vi "Init.vi"(11 "AllObjs[]":refnum<vi>[](array[refnum])) -> (1 "Ball Ref":cluster{refnum<vi>, "PaneColor":u32}[](array[cluster]), 2 "Array 2":refnum<vi>[](array[refnum]), 3 "Array":i32[](array[numeric]))   [LabVIEW 2014]
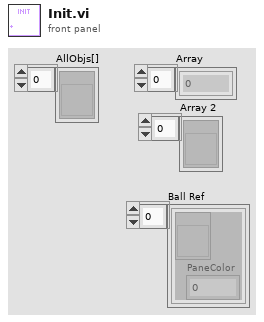
[diagram p1: front panel]
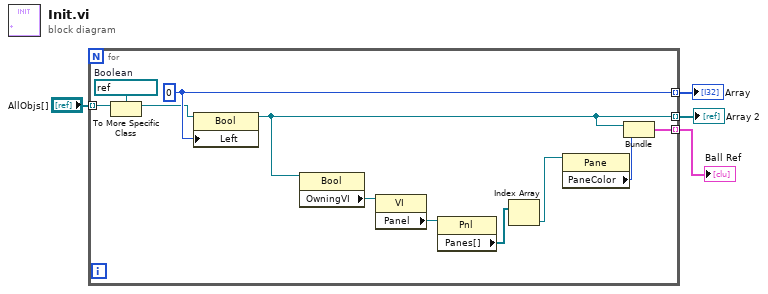
[diagram p0: block diagram]
diagram:
  n1 = for {
    tunnel: "AllObjs[]" -> [w14] mode=indexing
    tunnel: [w15] -> w4 mode=indexing
    tunnel: [w7] -> w2 mode=indexing
    tunnel: [w5] -> w1 mode=indexing
    w13 = refnum<vi> refnum  # Boolean
    w15 = 0 ("y")
    n2 = To More Specific Class(target class=w13, reference=w14) -> (specific class reference=w12:refnum<vi>)  [unwired: 1 in, 1 out]
    n3 = property class="Bool"(reference=w12, "Left"=w15) -> (reference out=w7:refnum<vi>)  [unwired: 1 in, 1 out]
    n4 = property class="Bool"(reference=w7) -> ("OwningVI"=w11:refnum<vi>)  [unwired: 1 in, 2 out]
    n5 = property class="VI"(reference=w11) -> ("Panel"=w10:refnum<vi>)  [unwired: 1 in, 2 out]
    n6 = property class="Pnl"(reference=w10) -> ("Panes[]"=w9:refnum<vi>[])  [unwired: 1 in, 2 out]
    n7 = Index Array(array=w9) -> (element=w8:refnum<vi>)  [unwired: 1 in]
    n8 = property class="Pane"(reference=w8) -> ("PaneColor"=w6:u32)  [unwired: 1 in, 2 out]
    n9 = Bundle(w7, "PaneColor"=w6) -> (w5:cluster{refnum<vi>, "PaneColor":u32})  [unwired: 1 in]
  }
  "Array" <- w4
  "Array 2" <- w2
  "Ball Ref" <- w1
